vi "Configure_Measurement.vi"(1 "DLL-Path":path, 2 "instanceHandle":u32, 3 "Error In":errorcluster caption="Fehler (Eingang, kein Fehler)") -> (0 "Fehler (Ausgang)":errorcluster)   [LabVIEW 2016]
uses:
  Utility/Global_Sensor.vi
  Program Files/MicroEpsilon/MEDAQLib-3.2.3.19901/Samples/LabView/MEDAQLib/MEDAQLib.lvlib
panel:
  out "ShutterTime Error":i32
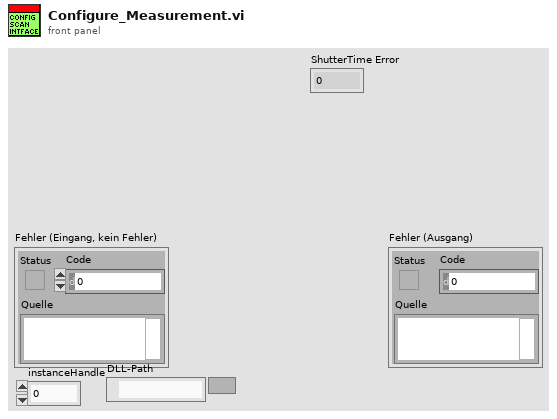
[diagram p1: front panel]
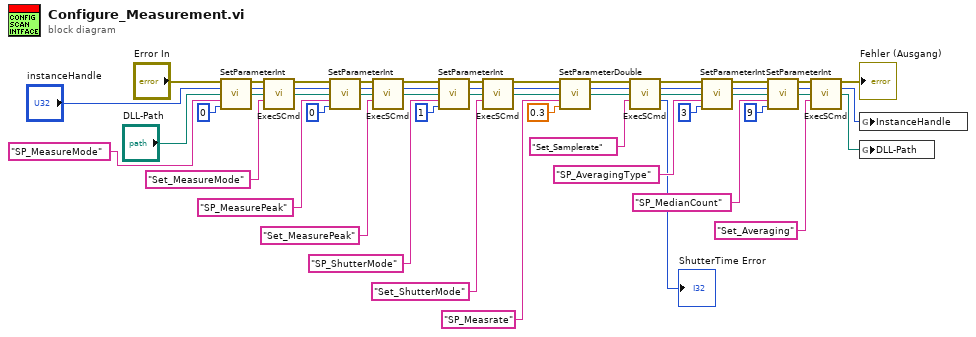
[diagram p0: block diagram]
diagram:
  n1 = call "SetParameterInt.vi"("Fehler (Eingang, kein Fehler)"="Error In", "instanceHandle"="instanceHandle", "DLL-Path"="DLL-Path", "paramName"="SP_MeasureMode", "paramValue"=0) -> ("Fehler (Ausgang)"=w54:errorcluster, "instanceHandle"=w53:u32, "DLL-Path"=w52:path)  [unwired: 7 in, 1 out]
  n2 = call "ExecSCmd.vi"("Fehler (Eingang, kein Fehler)"=w54, "instanceHandle"=w53, "DLL-Path"=w52, "sensorCommand"="Set_MeasureMode") -> ("Fehler (Ausgang)"=w21:errorcluster, "instanceHandle"=w20:u32, "DLL-Path"=w19:path)  [unwired: 8 in, 1 out]
  n3 = call "SetParameterInt.vi"("Fehler (Eingang, kein Fehler)"=w21, "instanceHandle"=w20, "DLL-Path"=w19, "paramName"="SP_MeasurePeak", "paramValue"=0) -> ("Fehler (Ausgang)"=w42:errorcluster, "instanceHandle"=w41:u32, "DLL-Path"=w40:path)  [unwired: 7 in, 1 out]
  n4 = call "ExecSCmd.vi"("Fehler (Eingang, kein Fehler)"=w42, "instanceHandle"=w41, "DLL-Path"=w40, "sensorCommand"="Set_MeasurePeak") -> ("Fehler (Ausgang)"=w24:errorcluster, "instanceHandle"=w23:u32, "DLL-Path"=w22:path)  [unwired: 8 in, 1 out]
  n5 = call "SetParameterInt.vi"("Fehler (Eingang, kein Fehler)"=w24, "instanceHandle"=w23, "DLL-Path"=w22, "paramName"="SP_ShutterMode", "paramValue"=1) -> ("Fehler (Ausgang)"=w30:errorcluster, "instanceHandle"=w29:u32, "DLL-Path"=w28:path)  [unwired: 7 in, 1 out]
  n6 = call "ExecSCmd.vi"("Fehler (Eingang, kein Fehler)"=w30, "instanceHandle"=w29, "DLL-Path"=w28, "sensorCommand"="Set_ShutterMode") -> ("Fehler (Ausgang)"=w9:errorcluster, "instanceHandle"=w8:u32, "DLL-Path"=w7:path)  [unwired: 8 in, 1 out]
  n7 = call "SetParameterDouble.vi"("Fehler (Eingang, kein Fehler)"=w9, "instanceHandle"=w8, "DLL-Path"=w7, "paramName"="SP_Measrate", "paramValue"=0.3) -> ("Fehler (Ausgang)"=w36:errorcluster, "instanceHandle"=w35:u32, "DLL-Path"=w34:path)  [unwired: 7 in, 1 out]
  n8 = call "ExecSCmd.vi"("Fehler (Eingang, kein Fehler)"=w36, "instanceHandle"=w35, "DLL-Path"=w34, "sensorCommand"="Set_Samplerate") -> ("Fehler (Ausgang)"=w3:errorcluster, "instanceHandle"=w2:u32, "DLL-Path"=w1:path, "ERR_CODE"=→"ShutterTime Error":i32)  [unwired: 8 in]
  n9 = call "SetParameterInt.vi"("Fehler (Eingang, kein Fehler)"=w3, "instanceHandle"=w2, "DLL-Path"=w1, "paramName"="SP_AveragingType", "paramValue"=3) -> ("Fehler (Ausgang)"=w16:errorcluster, "instanceHandle"=w15:u32, "DLL-Path"=w14:path)  [unwired: 7 in, 1 out]
  n10 = call "SetParameterInt.vi"("Fehler (Eingang, kein Fehler)"=w16, "instanceHandle"=w15, "DLL-Path"=w14, "paramName"="SP_MedianCount", "paramValue"=9) -> ("Fehler (Ausgang)"=w13:errorcluster, "instanceHandle"=w12:u32, "DLL-Path"=w11:path)  [unwired: 7 in, 1 out]
  n11 = call "ExecSCmd.vi"("Fehler (Eingang, kein Fehler)"=w13, "instanceHandle"=w12, "DLL-Path"=w11, "sensorCommand"="Set_Averaging") -> ("Fehler (Ausgang)"=→"Fehler (Ausgang)":errorcluster, "instanceHandle"=w6:u32, "DLL-Path"=w5:path)  [unwired: 8 in, 1 out]
  n12 = global write "Global_Sensor.vi" "InstanceHandle"(w6) -> ()
  n13 = global write "Global_Sensor.vi" "DLL-Path"(w5) -> ()
